vi "MathScript Fundamentals.vi"(11 "x":dbl[](array[numeric])=[1.0, 2.0, 3.0]) -> (0 "error out":errorcluster, 1 "y(1) in MathScript Node":dbl, 2 "y(1) in LabVIEW":dbl, 3 "y = x.^2":dbl[](array[numeric]))   [LabVIEW 2012]
doc: "This example shows: \na) How to use a script in a MathScript Node*; \nb) LabVIEW arrays are zero-indexed, while arrays in the MathScript Node are one-indexed; \nc) Many standard text-based math functions are available using the MathScript Node.\n\nInstructions:\n1) Run VI.\n2) Observe the outputs and their corresponding descriptions\n3) Look at the block diagram for more documentation"
uses:
  <vilib>/imath/engines/lvmath2/RunTimeEngine/ErrorHandling/NIMS_Finalize Error.vi
  <vilib>/imath/engines/lvmath2/RunTimeEngine/NodeEndStatement/NIMS_NodeEndStatement_Output.vi
  <instcachedir>/0/NIMS_NodeEndStatement_Output_53EC0D466D134D7ABD903AC30B43404B.lvgen/NIMS_NodeEndStatement_Output_53EC0D466D134D7ABD903AC30B43404B_001.vi
  <instcachedir>/0/NIMS_NodeEndStatement_Output_53EC0D466D134D7ABD903AC30B43404B.lvgen/NIMS_NodeEndStatement_Output_53EC0D466D134D7ABD903AC30B43404B_005.vi
  <vilib>/imath/engines/lvmath2/RunTimeEngine/VariableToken/Read/NIMS_Get Elements - RV(_) - Check.vi
  <instcachedir>/0/NIMS_Get Elements - RV(_) - Check_09E565EE58C54071A799578B82C9999A.lvgen/NIMS_Get Elements - RV(_) - Check_09E565EE58C54071A799578B82C9999A_000.vi
  <vilib>/imathl/engines/lvmath/Functions/Error Handling/Create Error.vi
  <vilib>/imath/engines/lvmath2/RunTimeEngine/BuiltInFunctions/dot/NIMS_dot(GV,GV).vi
  <instcachedir>/0/NIMS_dot(GV,GV)_B9FAA411F4494E9B94D442721014A3FA.lvgen/NIMS_dot(GV,GV)_B9FAA411F4494E9B94D442721014A3FA_000.vi
  <vilib>/imath/engines/lvmath2/RunTimeEngine/ErrorHandling/NIMS_Error From Error Code.vi
panel:
  out "Dot Product":dbl
  # "This example shows: \na) How to use a script in a MathScript Node*; \nb) LabVIEW arrays are zero-indexed, while arrays in the MathScript Node are one-indexed; \nc) Many standard text-based math functions are available using the MathScript Node.\n\nInstructions:\n1) Run VI.\n2) Observe the outputs and their corresponding descriptions\n3) Look at the block diagram for more documentation"
  # "x is array used as an input by\n the MathScript Node\n\n(a) y is generated by squaring x element by element. \nThis operation is performed in the MathScript Node. \nRefer to the Block Diagram for details on using the node.\n\n(b) Arrays in LabVIEW are zero-indexed. \nThus, y(1) is the second element of y.\n\nHowever, inside of the MathScript Node, \nindexing begins with 1, thus y(1) is the first element of y.\n\n(c) The MathScript Node supports many standard \ntextual math functions including Dot and Cross."
  # "*Scripts can also be run \ninteractively in the MathScript \nWindow. Select MathScript \nWindow from the Tools menu."
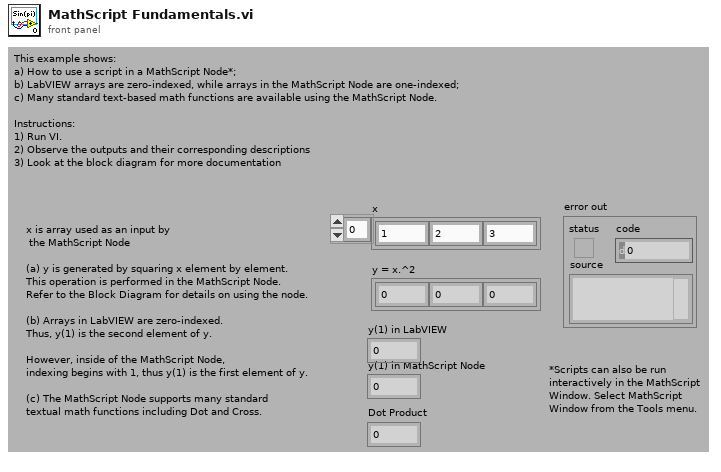
[diagram p1: front panel]
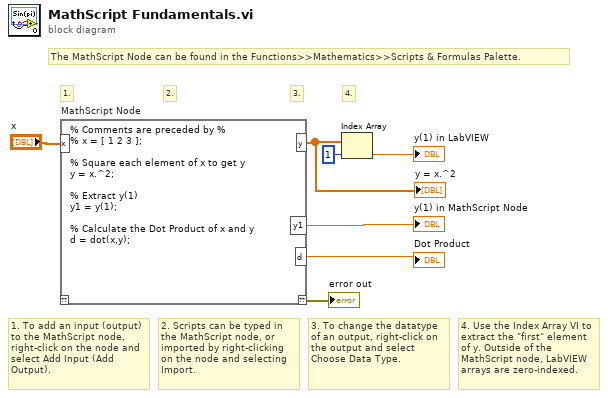
[diagram p0: block diagram]
diagram:
  # "4."
  # "4. Use the Index Array VI to extract the \"first\" element of y. Outside of the MathScript node, LabVIEW arrays are zero-indexed."
  # "The MathScript Node can be found in the Functions>>Mathematics>>Scripts & Formulas Palette."
  # "2. Scripts can be typed in the MathScript node, or imported by right-clicking on the node and selecting Import."
  # "3."
  # "2."
  # "1."
  # "1. To add an input (output) to the MathScript node, right-click on the node and select Add Input (Add Output)."
  # "3. To change the datatype of an output, right-click on the output and select Choose Data Type."
  n1 = mathscript code="% Comments are preceded by %\n% x = [ 1 2 3 ];\n\n% Square each element of x to get y\ny = x.^2;\n\n% Extract y(1)\ny1 = y(1);\n\n% Calculate the Dot Product of x and y\nd = dot(x,y);"("x"="x") -> ("??"=→"error out":errorcluster, "y"=w5:dbl[], "y1"=→"y(1) in MathScript Node":dbl, "d"=→"Dot Product":dbl)  [unwired: 1 in]
  "y = x.^2" <- w5
  n2 = Index Array "Index Array"(array=w5, index=1) -> (element=→"y(1) in LabVIEW":dbl)
